vi "get Last Error Addr.vi"(11 "cycloneHandle":u32) -> (3 "function return":u32)   [LabVIEW 2021, in "CycloneControlSDK.lvlib"]
doc: "extern \"C\" uint32_t _cdecl getLastErrorAddr(uint32_t cycloneHandle);"
uses:
  CycloneControlSDK.lvlib
  CycloneControlSDK_64.dll
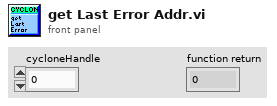
[diagram p1: front panel]
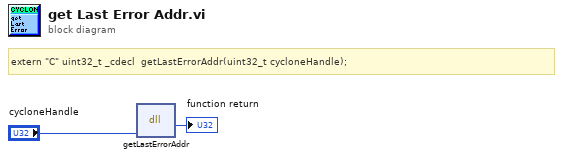
[diagram p0: block diagram]
diagram:
  # "extern \"C\" uint32_t _cdecl  getLastErrorAddr(uint32_t cycloneHandle);"
  n1 = dll-call lib="C:/PEMicro/cyclone/cycloneControl/controlsdk/examples/labview2018/user.lib/CycloneControlSDK/CycloneControlSDK_64.dll" fn="getLastErrorAddr"("cycloneHandle"="cycloneHandle") -> ("return type"=→"function return":u32)  [unwired: 4 in, 2 out]
